vi "Manage Score.vi"(11 "Game Board in":refnum<class "Game Board.lvclass">) -> (3 "Game Board out":refnum<class "Game Board.lvclass">)   [LabVIEW 2024, in "Game Board.lvclass"]
doc: "MIT Licence\nCopyright (c) 2024 David Grollier"
uses:
  Game Board.lvclass
  Game Board.lvclass/Game Board.ctl
  Game Componants.lvclass/Game Componants.ctl
  Game Board Component/Game Board Component.lvclass
  Game Componants.lvclass
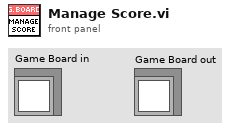
[diagram p1: front panel]
types:
  T1 = map{string, refnum<class "Game Board Component.lvclass">}
  T2 = typedef "Coordinates.ctl" = cluster{"x":dbl, "y":dbl}
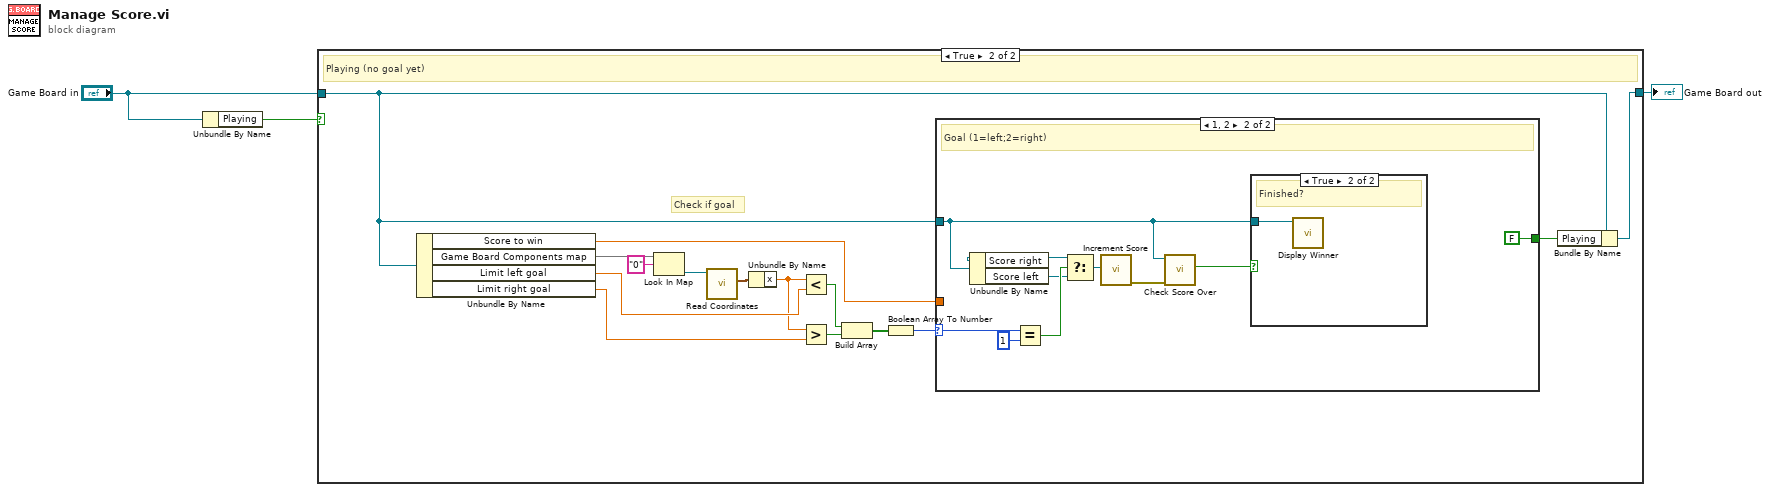
[diagram p0: block diagram]
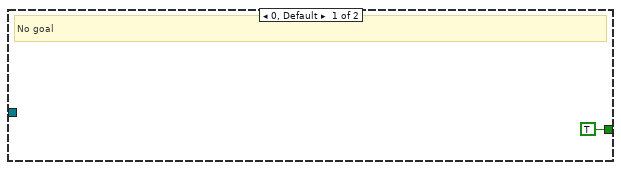
[diagram p3: hidden frame]
diagram:
  n1 = Unbundle By Name("Game Board in") -> ("Playing"=w1:bool)
  n2 = case shown="True" w1 {
    tunnel: [w4 w7] -> w3
    tunnel: "Game Board in" -> [w4 w5]
    frame False {
      # "Not playing (already scored)"
    }
    frame True {
      # "Check if goal"
      # "Playing (no goal yet)"
      n3 = Unbundle By Name(w5) -> ("Score to win"=w8:dbl, "Game Board Components map"=w19:T1, "Limit left goal"=w15:dbl, "Limit right goal"=w14:dbl)
      n4 = Look In Map(map=w19, key="0") -> (value=w17:refnum<class "Game Board Component.lvclass">)  [unwired: 1 in, 1 out]
      n5 = call "Read Coordinates.vi"("Game Componants in"=w17) -> ("Coordinates"=w16:T2)  [unwired: 10 in]
      n6 = Unbundle By Name(w16) -> ("x"=w13:dbl)
      n7 = Less?(x=w13, y=w15) -> (x < y?=w12:bool)
      n8 = Greater?(x=w13, y=w14) -> (0:w11:bool)
      n9 = Build Array(w12, w11) -> (w10:bool[])
      n10 = Boolean Array To Number(Boolean array=w10) -> (number=w9:u32)
      n11 = case shown="1, 2" w9 {
        selector: w9 -> [_ w28]
        tunnel: w5 -> [_ w22]
        tunnel: w8 -> [_ _]
        tunnel: [TRUE ("Playing") FALSE ("Playing")] -> w6
        frame 0, Default {
          # "No goal"
        }
        frame 1, 2 {
          # "Goal (1=left;2=right)"
          n12 = Unbundle By Name(w22) -> ("Score right"=w26:refnum<vi>, "Score left"=w25:refnum<vi>)
          n13 = Equal?(x=w28, y=u32 1) -> (x = y?=w27:bool)
          n14 = Select(t=w26, s=w27, f=w25) -> (s? t:f=w24:refnum<vi>)
          n15 = call "Increment Score.vi"("Score ref in"=w24) -> ("error out"=w30:errorcluster)  [unwired: 10 in]
          n16 = call "Check Score Over.vi"("error in (no error)"=w30, "Game Board in"=w22) -> ("Score over?"=w23:bool)  [unwired: 9 in]
          n17 = case shown="True" w23 {
            tunnel: w22 -> [_ w31]
            frame False {
            }
            frame True {
              # "Finished?"
              n18 = call "Display Winner.vi"("Game Board in"=w31) -> ()  [unwired: 11 in]
            }
          }
        }
      }
      n19 = Bundle By Name(cluster=w5, "Playing"=w6) -> (w7:refnum<class "Game Board.lvclass">)
    }
  }
  "Game Board out" <- w3
